vi "Populate Triggerable Frames with Messages.vi"(8 "error in":errorcluster, 10 "transmitted messages":T2[](array[typedef]) {"Timestamp Channel Handle" format="%.0x"; "Message Section Handle" format="%.0x"; "Parameter Channel Handles" format="%.0x"}, 11 "port":T3 format="%.0x") -> (0 "error out":errorcluster, 2 "trigger channels":T3[](array[typedef]) format="%.0x", 3 "triggerable frames":T1[](array[typedef]) {"Acyclic Messages"."Timestamp Channel Handle" format="%.0x"; "Acyclic Messages"."Message Section Handle" format="%.0x"; "Acyclic Messages"."Parameter Channel Handles" format="%.0x"})   [LabVIEW 2020, in "AIM MIL-STD-1553 Engine.lvlib" / "Implementation.lvlib" / "Tx Acyclic Execution Unit.lvclass"]
uses:
  Tx Acyclic Execution Unit.lvclass
  Scripting/AIM MIL-STD-1553 Scripting.lvlib
  <vilib>/NI VeriStand/Custom Device API/Custom Device Item Ref.ctl
  <vilib>/NI VeriStand/Custom Device API/Custom Device API.lvlib
  Shared/Direction.ctl
  Shared/Parameter Definition.ctl
  Custom Device/Compiled Message.ctl
  Custom Device/Custom Device.lvlib
  Triggerable Frame.ctl
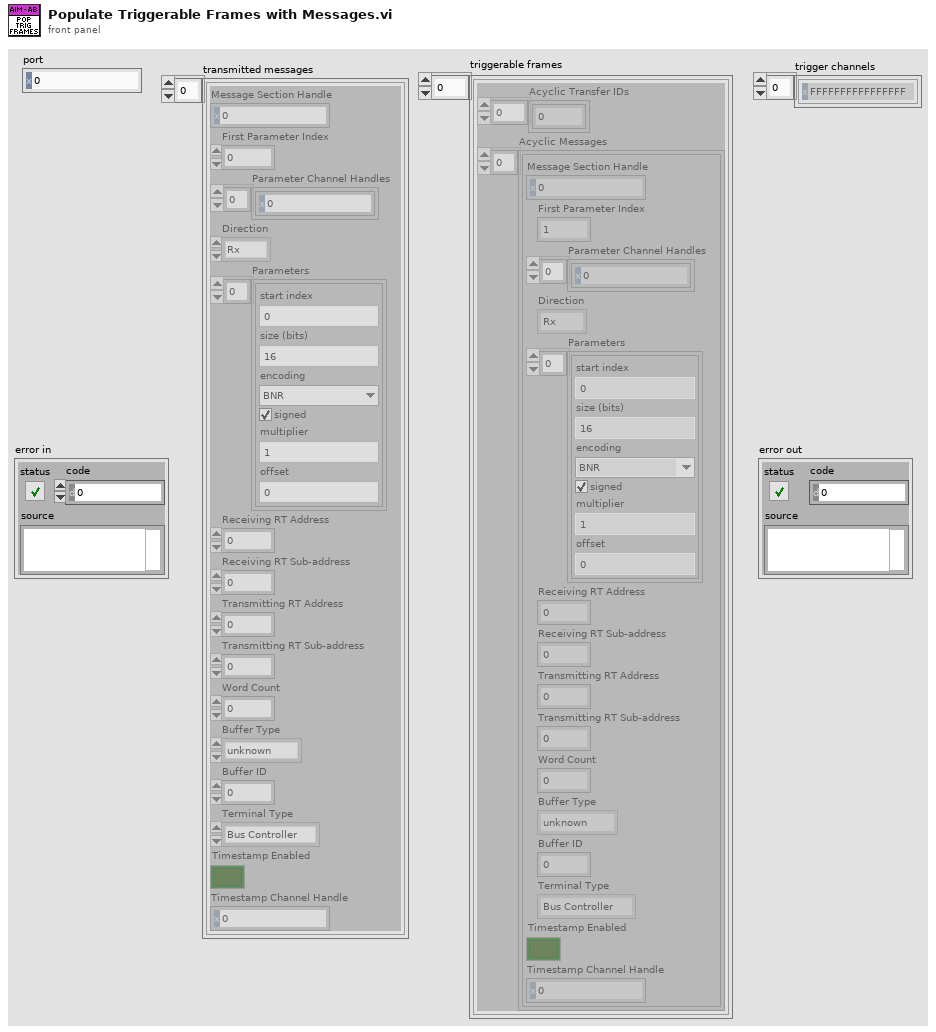
[diagram p1: front panel]
types:
  T1 = typedef "AIM MIL-STD-1553 Engine.lvlib/Implementation.lvlib/Tx Acyclic Execution Unit.lvclass/Triggerable Frame.ctl" = cluster{"Acyclic Transfer IDs":u16[], "Acyclic Messages":T2[]}
  T2 = typedef "AIM MIL-STD-1553 Engine.lvlib/Custom Device.lvlib/Compiled Message.ctl" = cluster{"Message Section Handle":T3, "First Parameter Index":i32, "Parameter Channel Handles":T3[], "Direction":T4, "Parameters":T5[], "Receiving RT Address":u8, "Receiving RT Sub-address":u8, "Transmitting RT Address":u8, "Transmitting RT Sub-address":u8, "Word Count":u8, "Buffer Type":enum16{"unknown", "BC Message Buffer", "RT Message Buffer"}, "Buffer ID":u16, "Terminal Type":enum16{"Bus Controller", "Remote Terminal"}, "Timestamp Enabled":bool, "Timestamp Channel Handle":T3}
  T3 = typedef "Custom Device API.lvlib/Custom Device Item Ref.ctl" = u64
  T4 = typedef "Direction.ctl" = enum16{"Rx", "Tx"}
  T5 = typedef "Parameter Definition.ctl" = cluster{"start index":i32, "size (bits)":i32, "encoding":enum16{"BNR", "BCD", "Discrete"}, "signed":bool, "multiplier":dbl, "offset":dbl}
  T6 = typedef "Acyclic Frame Definition.ctl" = cluster{"name":string, "messages":string[]}
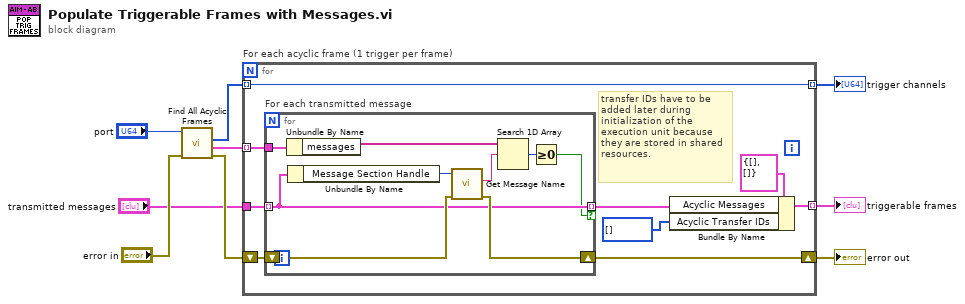
[diagram p0: block diagram]
diagram:
  n1 = call "Find All Acyclic Frames.vi"("error in"="error in", "port"="port") -> ("error out"=w6:errorcluster, "acyclic frames"=w2:T6[], "acyclic frame triggers"=w1:T3[])  [unwired: 6 in, 1 out]
  n2 = for "For each acyclic frame (1 trigger per frame)" {
    shift-right: [w17] -> w7
    shift-left: w6 -> [w18]
    tunnel: w2 -> [w15] mode=indexing
    tunnel: "transmitted messages" -> [w16]
    tunnel: [w12] -> w4 mode=indexing
    tunnel: [w10] -> w3 mode=indexing
    tunnel: w1 -> [w10] mode=indexing
    # "transfer IDs have to be added later during initialization of the execution unit because they are stored in shared resources."
    n3 = for "For each transmitted message" {
      shift-right: [w25] -> w17
      shift-left: w18 -> [w26]
      tunnel: w16 -> [w20] mode=indexing
      tunnel: w15 -> [w24]
      tunnel: [w20] -> w13 mode=indexing if=w19
      n4 = Unbundle By Name(w24) -> ("messages"=w23:string[])
      n5 = Unbundle By Name(w20) -> ("Message Section Handle"=w27:T3)
      n6 = call "Get Message Name.vi"("error in"=w26, "message or subaddress"=w27) -> ("error out"=w25:errorcluster, "name"=w22:string)  [unwired: 6 in, 2 out]
      n7 = Search 1D Array(1D array=w23, element=w22) -> (index of element=w21:i32)  [unwired: 1 in]
      n8 = Greater Or Equal To 0?(x=w21) -> (x >= 0?=w19:bool)
    }
    n9 = Bundle By Name(cluster=T1 {"Acyclic Transfer IDs"=[], "Acyclic Messages"=[]} ("triggerable frames"), "Acyclic Messages"=w13, "Acyclic Transfer IDs"=u16[] []) -> (w12:T1)
  }
  "error out" <- w7
  "trigger channels" <- w3
  "triggerable frames" <- w4
